vi "CustomDebugData.vi"(0 "Subroutine":string, 11 "error in (no error)":errorcluster) -> (4 "DebugInfo":string, 15 "error out":errorcluster)   [LabVIEW 2021, in "Event Logger.lvlib"]
uses:
  Event Logger.lvlib
  <vilib>/Utility/error.llb/DialogType.ctl
  Migrator/Migrator Reusables/Migrator Reusables.lvlib
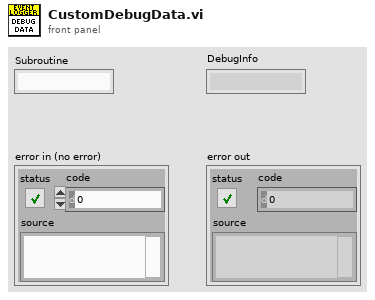
[diagram p1: front panel]
types:
  T1 = typedef "DialogType.ctl" = u16
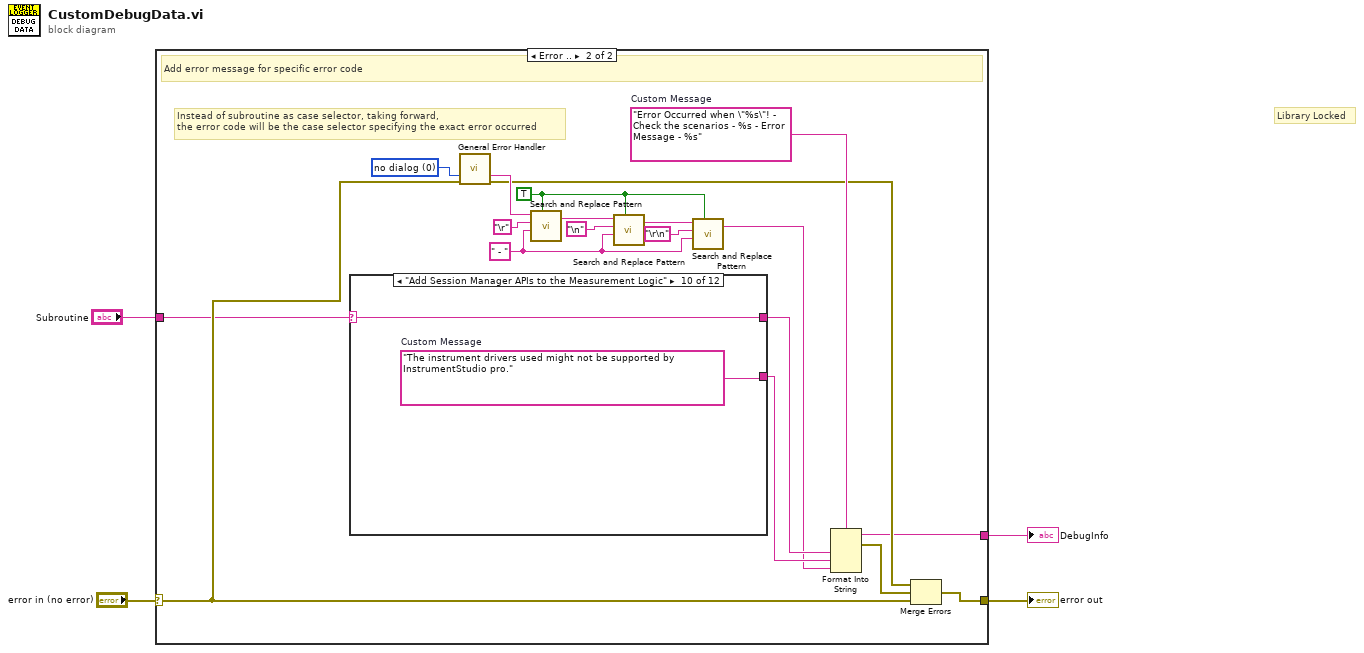
[diagram p0: block diagram]
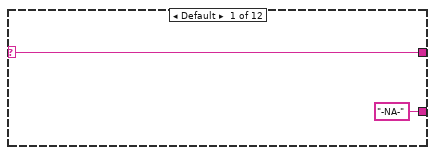
[diagram p3: hidden frame]
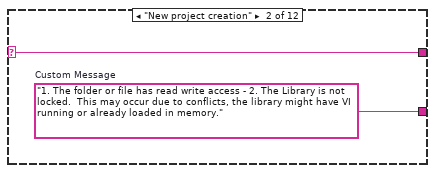
[diagram p4: hidden frame]
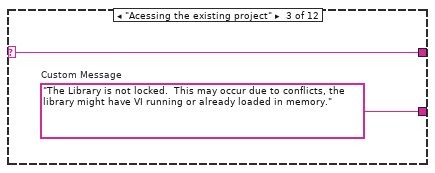
[diagram p5: hidden frame]
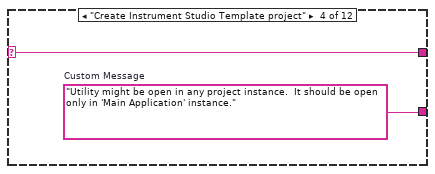
[diagram p6: hidden frame]
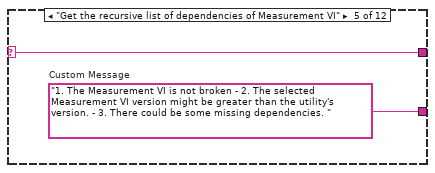
[diagram p7: hidden frame]
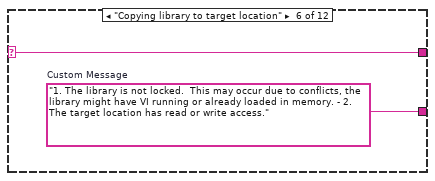
[diagram p8: hidden frame]
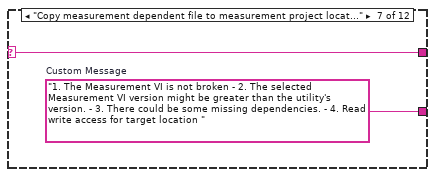
[diagram p9: hidden frame]
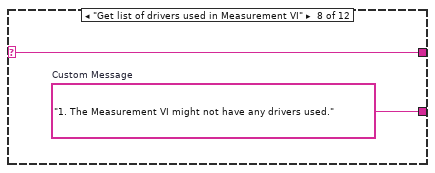
[diagram p10: hidden frame]
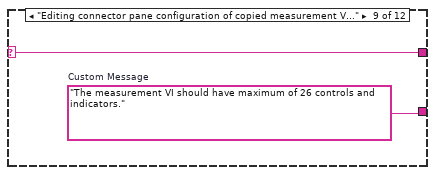
[diagram p11: hidden frame]
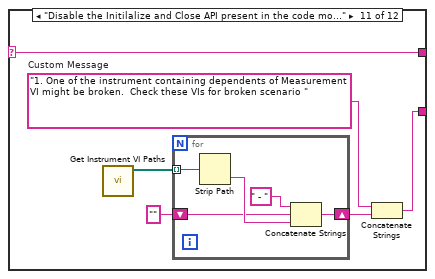
[diagram p12: hidden frame]
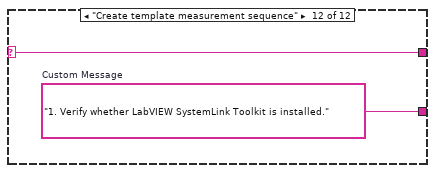
[diagram p13: hidden frame]
diagram:
  # "Library Locked"
  n1 = case shown="Error .." "error in (no error)" {
    selector: "error in (no error)" -> [w5 w7]
    tunnel: [w5 w12] -> w4
    tunnel: [_ w9] -> w2
    tunnel: "Subroutine" -> [_ w6]
    frame No Error {
    }
    frame Error {
      w8 = TRUE ("replace all? (F)")
      w16 = "Error Occurred when \"%s\"! - Check the scenarios - %s - Error Message - %s"  # Custom Message
      w24 = " - "
      w17 = T1 0 items=["no dialog", "OK message", "continue or stop message", "OK message + warnings", "continue/stop + warnings"] ("type of dialog (OK msg:1)")
      # "Instead of subroutine as case selector, taking forward, \nthe error code will be the case selector specifying the exact error occurred"
      # "Add error message for specific error code"
      n2 = case shown="\"Add Session Manager APIs to the Measurement Logic\"" w6 {
        selector: w6 -> [w26 w28 w30 w31 w34 w36 w38 w40 w42 w44 w50 w57]
        tunnel: [w26 w28 w30 w31 w34 w36 w38 w40 w42 w44 w50 w57] -> w15
        tunnel: ["-NA-" ("Custom Message") w27 w29 w32 w33 w35 w37 w39 w41 w43 w45 w56] -> w14
        frame Default {
        }
        frame "New project creation" {
          w27 = "1. The folder or file has read write access - 2. The Library is not locked.  This may occur due to conflicts, the library might have VI running or already loaded in memory."  # Custom Message
        }
        frame "Acessing the existing project" {
          w29 = "The Library is not locked.  This may occur due to conflicts, the library might have VI running or already loaded in memory."  # Custom Message
        }
        frame "Create Instrument Studio Template project" {
          w32 = "Utility might be open in any project instance.  It should be open only in 'Main Application' instance."  # Custom Message
        }
        frame "Get the recursive list of dependencies of Measurement VI" {
          w33 = "1. The Measurement VI is not broken - 2. The selected Measurement VI version might be greater than the utility's version. - 3. There could be some missing dependencies. "  # Custom Message
        }
        frame "Copying library to target location" {
          w35 = "1. The library is not locked.  This may occur due to conflicts, the library might have VI running or already loaded in memory. - 2. The target location has read or write access."  # Custom Message
        }
        frame "Copy measurement dependent file to measurement project location" {
          w37 = "1. The Measurement VI is not broken - 2. The selected Measurement VI version might be greater than the utility's version. - 3. There could be some missing dependencies. - 4. Read write access for target location "  # Custom Message
        }
        frame "Get list of drivers used in Measurement VI" {
          w39 = "1. The Measurement VI might not have any drivers used."  # Custom Message
        }
        frame "Editing connector pane configuration of copied measurement VI" {
          w41 = "The measurement VI should have maximum of 26 controls and indicators."  # Custom Message
        }
        frame "Add Session Manager APIs to the Measurement Logic" {
          w43 = "The instrument drivers used might not be supported by InstrumentStudio pro."  # Custom Message
        }
        frame "Disable the Initilalize and Close API present in the code module" {
          w48 = "1. One of the instrument containing dependents of Measurement VI might be broken.  Check these VIs for broken scenario "  # Custom Message
          n3 = call "Get Instrument VI Paths.vi"() -> ("Instr VI Paths[]"=w46:path[])  [unwired: 10 in, 1 out]
          n4 = for {
            tunnel: w46 -> [w55] mode=indexing
            shift-right: [w51] -> w49
            shift-left: "" -> [w53]
            n5 = Strip Path(path=w55) -> (name=w54:string)  [unwired: 1 out]
            n6 = Concatenate Strings(" - " ("string"), w53, w54) -> (w51:string)
          }
          n7 = Concatenate Strings(w48, w49) -> (w45:string)
        }
        frame "Create template measurement sequence" {
          w56 = "1. Verify whether LabVIEW SystemLink Toolkit is installed."  # Custom Message
        }
      }
      n8 = call <vilib>:"General Error Handler.vi"("type of dialog (OK msg:1)"=w17, "error in (no error)"=w7) -> ("message"=w18:string, "error out"=w10:errorcluster)  [unwired: 9 in, 3 out]
      n9 = call <vilib>:"Search and Replace Pattern.vi"("string"=w18, "regular expression (\"\")"="\r", "replace string (\"\")"=w24, "replace all? (F)"=w8) -> ("result string"=w22:string)  [unwired: 1 in, 1 out]
      n10 = call <vilib>:"Search and Replace Pattern.vi"("string"=w22, "regular expression (\"\")"="\n", "replace string (\"\")"=w24, "replace all? (F)"=w8) -> ("result string"=w23:string)  [unwired: 1 in, 1 out]
      n11 = call <vilib>:"Search and Replace Pattern.vi"("string"=w23, "regular expression (\"\")"="\r\n", "replace string (\"\")"=w24, "replace all? (F)"=w8) -> ("result string"=w13:string)  [unwired: 1 in, 1 out]
      n12 = Format Into String(format string=w16, w15, w14, w13) -> (resulting string=w9:string, error out=w11:errorcluster)  [unwired: 2 in]
      n13 = Merge Errors(w10, w11, w7) -> (w12:errorcluster)
    }
  }
  "error out" <- w4
  "DebugInfo" <- w2
